vi "RSMA Receiver - 1 Channel.vi"() -> ()   [LabVIEW 2022 SP3]
panel:
  out "Decoded message":string
  out "Constellation Map":cdb[](graph)
  in  "Decode M2?":bool
  in  "Tab Control":enum32{"USRP Parameters", "Rx Info", "BER"}(tab)
  in  "USRP ControledParameters":T1={"Active Antenna"="RX2", "Gain (dB)"=0.0, "Carrier Frequency"=2400000000.0, "IQ Rate"=2000000.0, "Active channels"="0"} {"IQ Rate" format="%#_6p"; "Carrier Frequency" format="%#_6p"; "Gain (dB)" format="%#_6f"}
  in  "Device selection":refnum<k15>="RIO0"
  in  "Trigger level":dbl=0.01 format="%f"
  out "?":T2
  out "SIG valid?":bool
  out "Frequency offset":dbl
  out "Coerced Parameters":T3={"IQ Rate"=100000.0, "Carrier  Freq."=100000.0, "Gain"=0.0} {"Gain" format="%#_6f"; "Carrier  Freq." format="%#_6p"; "IQ Rate" format="%#_6p"}
  out "Error out":errorcluster
  in  "Expected message":string="ptua. At vero eos et accusam et justo duo dolores et ea rebum. Stet clita kasd gubergren, no sea takimata sanctus est Lorem ipsum dolor sit amet. Lore"
  in  "Record BER":bool
  in  "Refresh Button":bool
  out "Inst. BER":dbl format="%#_4g"
  out "No. Bits":dbl format="%#_6f"
  out "Acum. Err":dbl
  out "Acc. BER":dbl format="%#_4g"
  in  "error in (no error)":errorcluster
  # "RSMA Reeciever"
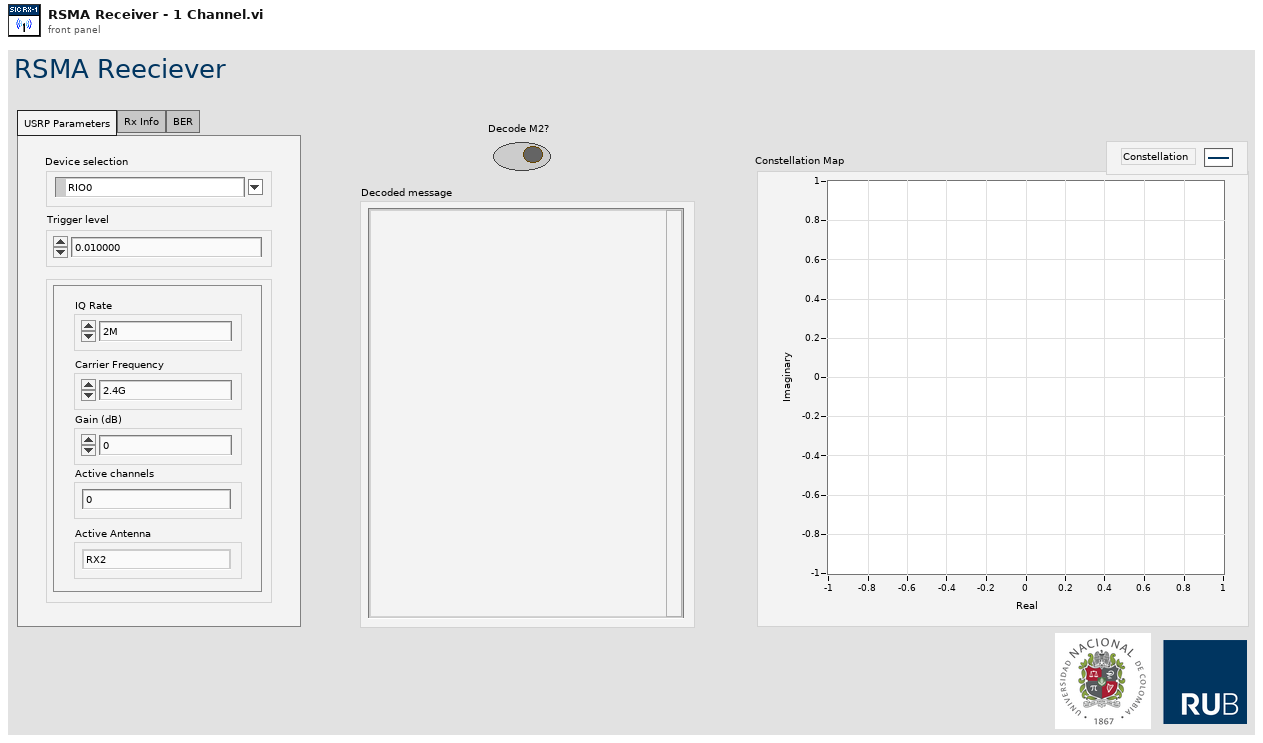
[diagram p1: front panel]
types:
  T1 = cluster{"Active Antenna":string, "Gain (dB)":dbl, "Carrier Frequency":dbl, "IQ Rate":dbl, "Active channels":string}
  T2 = cluster{"Modulation type":enum16{"QPSK(4QAM)", "64QAM", "16QAM", "BPSK"}, "BCC rate (k/n)":enum16{"1/2", "2/3", "3/4"}}
  T3 = cluster{"IQ Rate":dbl, "Carrier  Freq.":dbl, "Gain":dbl}
  T4 = cluster{"coerced IQ rate":dbl, "coerced carrier frequency":dbl, "coerced gain":dbl}
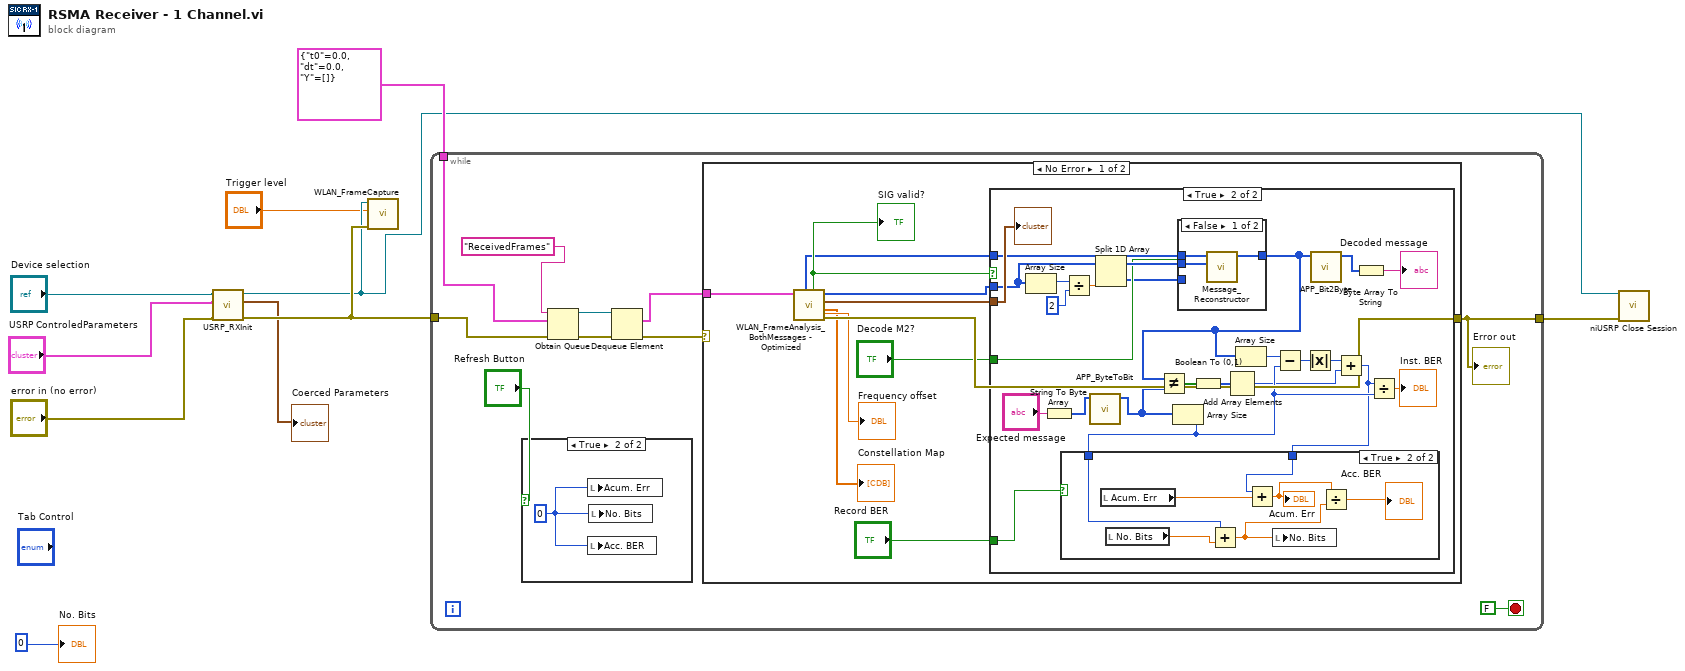
[diagram p0: block diagram]
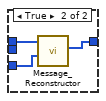
[diagram p4: hidden frame]
diagram:
  n1 = call "USRP_RXInit.vi"("device names"="Device selection", "USRP ControledParameters"="USRP ControledParameters", "error in (no error)"="error in (no error)") -> ("session handle out"=w6:refnum<k15>, "USRP CoercedParamters"=→"Coerced Parameters":T4, "error out"=w9:errorcluster)  [unwired: 5 in]
  n2 = call "WLAN_FrameCapture.vi"("error in (no error)"=w9, "Trigger level"="Trigger level", "session handle"=w6) -> ()  [unwired: 8 in]
  n3 = while {
    tunnel: w9 -> [w19]
    tunnel: cluster{"t0":dbl, "dt":dbl, "Y":cdb[]} {"t0"=0.0, "dt"=0.0, "Y"=[]} ("data") -> [w20]
    tunnel: [w13] -> w7
    stop <- FALSE stop-if-true
    n4 = case shown="True" "Refresh Button" {
      frame False {
      }
      frame True {
        w21 = 0
        n5 = local write "Acum. Err"(w21) -> ()
        n6 = local write "Acc. BER"(w21) -> ()
        n7 = local write "No. Bits"(w21) -> ()
      }
    }
    n8 = Obtain Queue(name (unnamed)="ReceivedFrames", element data type=w20, error in (no error)=w19) -> (queue out=w18:refnum<queue>, error out=w15:errorcluster)  [unwired: 2 in, 1 out]
    n9 = Dequeue Element(queue=w18, error in (no error)=w15) -> (element=w16:cluster{"t0":dbl, "dt":dbl, "Y":cdb[]}, error out=w17:errorcluster)  [unwired: 1 in, 2 out]
    n10 = case shown="No Error" w17 {
      selector: w17 -> [_ w70]
      tunnel: w16 -> [w29 _]
      tunnel: [w30 w70] -> w13
      frame No Error {
        n11 = call "WLAN_FrameAnalysis_BothMessages - Optimized.vi"("input cluster"=w29) -> ("error out"=w30:errorcluster, "Constellation"=→"Constellation Map":cdb[], "Modulation parameter"=w31:T2, "SC Bits"=w23:i8[], "Frequency offset"=→"Frequency offset":dbl, "SIG valid?"=w28:bool, "Base Bits"=w24:i8[])  [unwired: 4 in]
        "SIG valid?" <- w28
        n12 = case shown="True" w28 {
          tunnel: w31 -> [_ w56]
          tunnel: "Record BER" -> [_ w49]
          tunnel: w24 -> [_ w36]
          tunnel: w23 -> [_ w32]
          tunnel: "Decode M2?" -> [_ w35]
          frame False {
          }
          frame True {
            n13 = Array Size(array=w32) -> (size(s)=w39:i32)
            n14 = String To Byte Array(string="Expected message") -> (unsigned byte array=w48:u8[])
            n15 = Divide(x=w39, y=2) -> (x/y=w40:dbl)
            n16 = call "APP_ByteToBit.vi"("byte array"=w48) -> ("bit array"=w47:i8[])  [unwired: 9 in]
            n17 = Split 1D Array(array=w32, index=w40) -> (first subarray=w37:i8[], second subarray=w34:i8[])
            n18 = Array Size(array=w47) -> (size(s)=w43:i32)
            n19 = case shown="False" w35 {
              tunnel: [w59 w60] -> w38
              tunnel: w37 -> [w58 _]
              tunnel: w36 -> [w57 w61]
              tunnel: w34 -> [_ w62]
              frame False {
                n20 = call "Message_Reconstructor.vi"("Wp1"=w58, "Wc"=w57) -> ("W1"=w59:u8[])  [unwired: 8 in, 1 out]
              }
              frame True {
                n21 = call "Message_Reconstructor.vi"("Wp2"=w62, "Wc"=w61) -> ("W2"=w60:u8[])  [unwired: 8 in, 1 out]
              }
            }
            n22 = Not Equal?(x=w38, y=w47) -> (x != y?=w52:bool[])
            n23 = Boolean To (0,1)(Boolean=w52) -> (0, 1=w51:i16[])
            n24 = Add Array Elements(numeric array=w51) -> (sum=w42:i16)
            n25 = Array Size(array=w38) -> (size(s)=w46:i32)
            n26 = Subtract(x=w46, y=w43) -> (x-y=w45:i32)
            n27 = Absolute Value(x=w45) -> (abs(x)=w44:i32)
            n28 = call "APP_Bit2Byte.vi"("input bit stream"=w38) -> ("output byte stream"=w50:u8[])  [unwired: 10 in]
            n29 = Add(x=w44, y=w42) -> (x+y=w41:i32)
            n30 = case shown="True" w49 {
              tunnel: w43 -> [_ w68]
              tunnel: w41 -> [_ w66]
              frame False {
              }
              frame True {
                n31 = local read "Acum. Err"() -> (w67:dbl)
                n32 = local read "No. Bits"() -> (w69:dbl)
                n33 = Add(x=w68, y=w69) -> (x+y=w65:dbl)
                n34 = Add(x=w66, y=w67) -> (x+y=w64:dbl)
                "Acum. Err" <- w64
                n35 = local write "No. Bits"(w65) -> ()
                n36 = Divide(x=w64, y=w65) -> (x/y=→"Acc. BER":dbl)
              }
            }
            n37 = Byte Array To String(unsigned byte array=w50) -> (string=→"Decoded message":string)
            n38 = Divide(x=w41, y=w43) -> (x/y=→"Inst. BER":dbl)
            "?" <- w56
          }
        }
      }
      frame Error {
      }
    }
    "Error out" <- w13
  }
  n39 = call <instrlib>:"niUSRP Close Session.vi"("session handle"=w6, "error in (no error)"=w7) -> ()  [unwired: 13 in, 1 out]
  "No. Bits" <- 0
